vi "ge_EditCell.vi"(4 "HiLite":bool, 6 "Mod":bool, 7 "MeasType":T3, 8 "error in":errorcluster, 9 "Active Cell":T4, 10 "ge_DAQManDefinitions":T1, 11 "FP Ctrl":T2) -> (0 "error out":errorcluster, 1 "Discard?":bool)   [LabVIEW 2018]
uses:
  <vilib>/Utility/miscctls.llb/LVRowAndColumnTypeDef.ctl
  Custom Ctrls/ge_MeasType.ctl
  Custom Ctrls/ge_FPCtrlRefLabel.ctl
  Common/Controls/DAQMan Definitions.ctl
  Custom Ctls Table/ge_HdrInfo.ctl
  Custom Ctls Table/ge_GlblCtrls.ctl
  Custom Ctls Table/ge_ColType.ctl
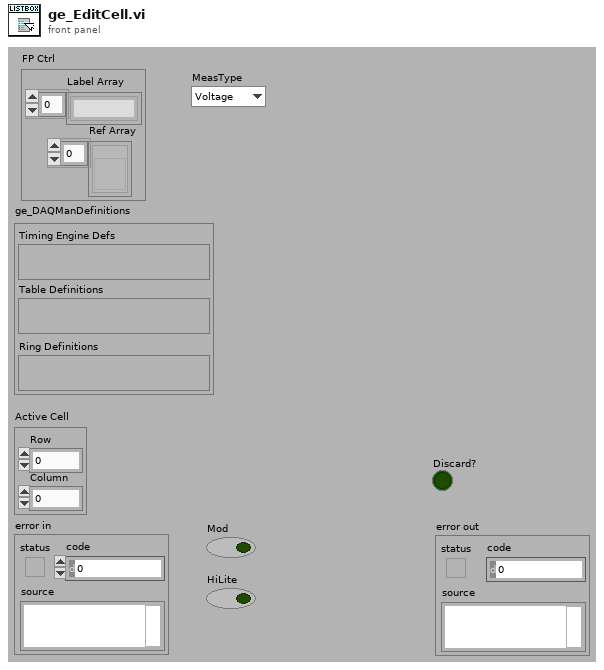
[diagram p1: front panel]
types:
  T1 = typedef "DAQMan Definitions.ctl" = cluster{"Timing Engine Defs":variant, "Table Definitions":variant, "Ring Definitions":variant}
  T2 = typedef "ge_FPCtrlRefLabel.ctl" = cluster{"Label Array":string[], "Ref Array":refnum<vi>[]}
  T3 = typedef "ge_MeasType.ctl" = enum16{"Voltage", "Frequency", "Tachometer", "Dynamic", "Thermocouple", "RTD", "Strain", "Current", "Resistance"}
  T4 = typedef "LVRowAndColumnTypeDef.ctl" = cluster{"Row":i32, "Column":i32}
  T5 = typedef "ge_HdrInfo.ctl" = cluster{"Hdr Width":i32, "Glbl Ctrl":T6}
  T6 = typedef "ge_GlblCtrls.ctl" = enum16{"Str0", "Bool0", "Bool1", "Int0", "Ring0", "Ring1", "Ring2", "Ring3", "Dbl0", "Dbl1", "Dbl2", "Dbl3", "Cal0", "Cal1", "Cal2", "None"}
  T7 = typedef "LVPositionTypeDef.ctl" = cluster{"Left":i32, "Top":i32}
  T8 = typedef "LVBoundsTypeDef.ctl" = cluster{"Width":u32, "Height":u32}
  T9 = typedef "ge_ColType.ctl" = enum16{"Volts", "Amps", "Ohms", "TermCfg", "WireCfg", "Coup", "Slope", "Iex", "CalUnits", "ThrmUnits", "ThrmType", "CJCSrc", "BrdgType", "Strn Mode", "RTDType"}
  T10 = typedef "HeaderNames.ctl" = enum16{"Channel", "Device", "Spacer", "Description", "MB", "Range", "Terminal", "Coupling", "Thresh (V)", "Pulse/Rev", "Slope", "Min EU", "Min RPM", "mV/EU", "Iex", "Temp Units", "Type", "CJC Src", "CJC Val", "Ro", "Wire Cfg", "Strain Mode", "Vex", "Bridge Type", "GF", "Gauge Res", "Poisson", "Lead Res", "Init Strain", "GAF", "Scale", "Offset", "Unit (EU)", "dB?", "dB Ref", "Cal Mag", "Cal Units", "Max Temp", "Min Temp", "Max Strain", "Min Strain"}
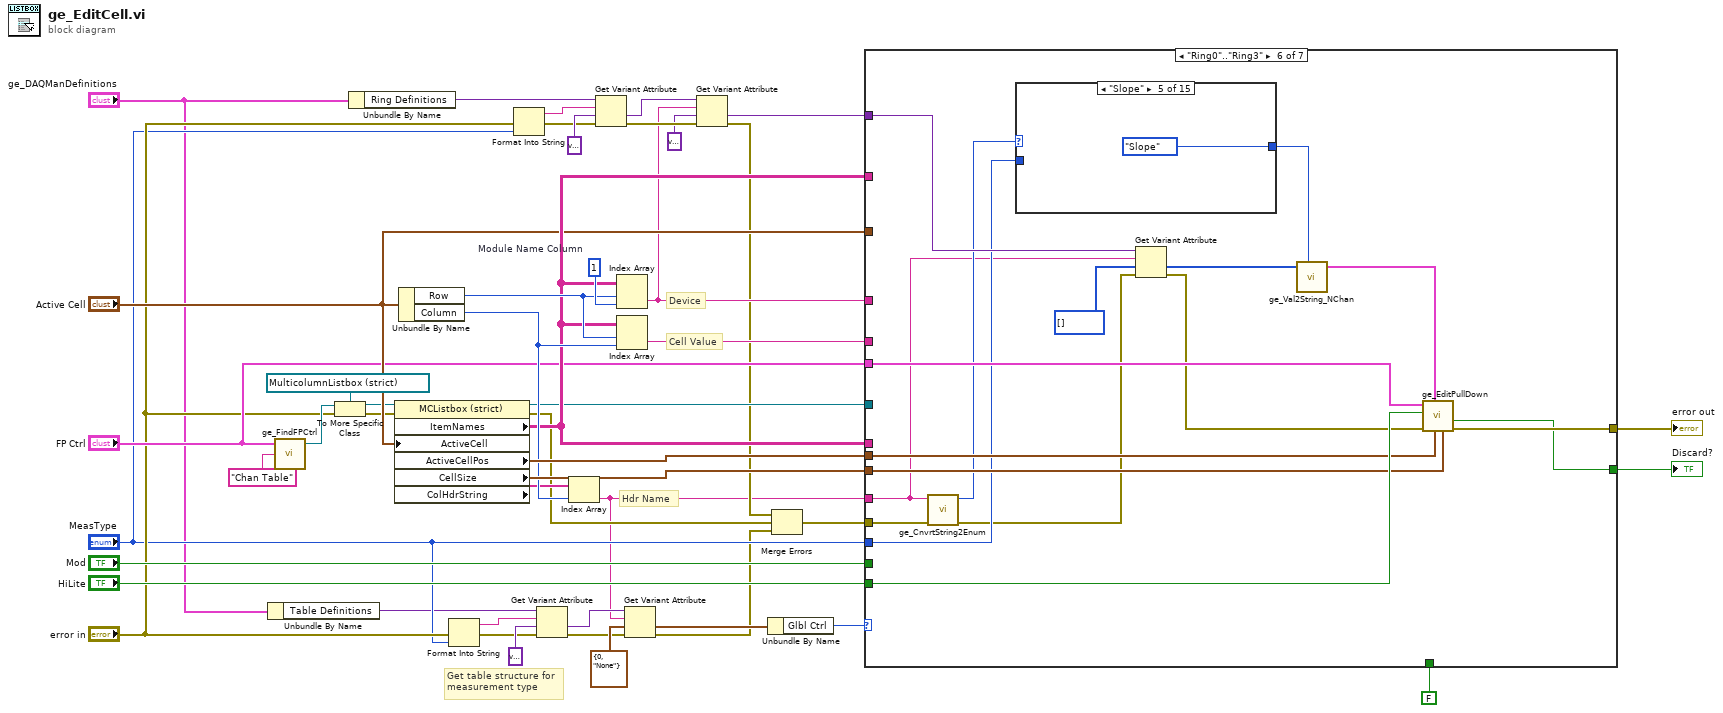
[diagram p0: block diagram]
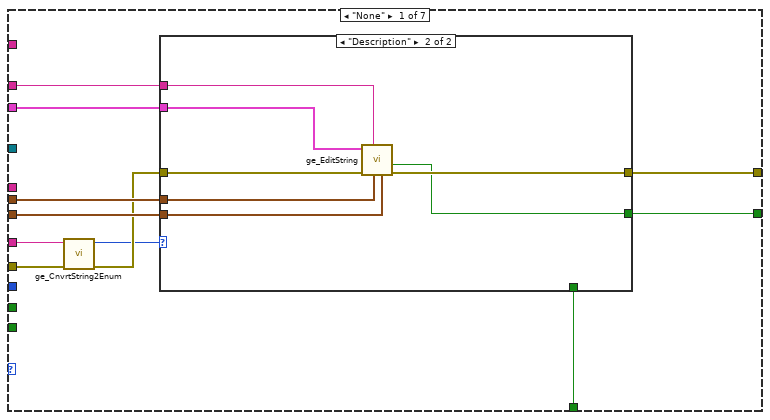
[diagram p2: hidden frame]
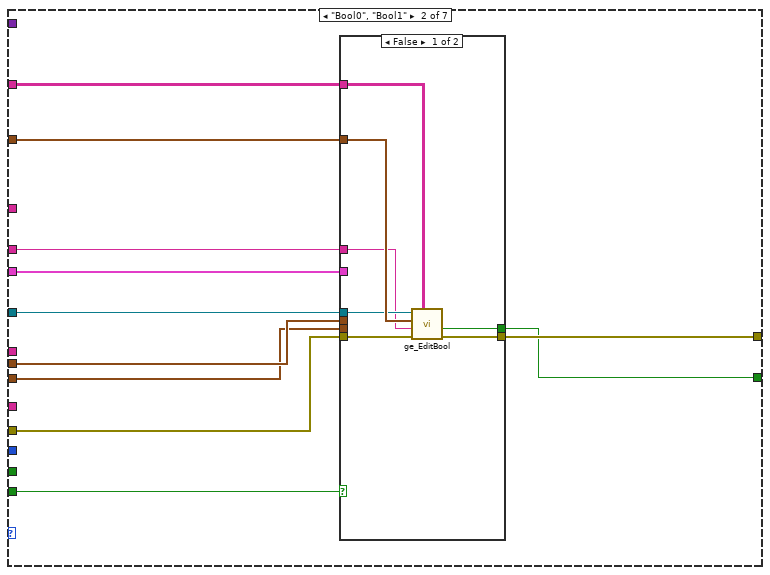
[diagram p4: hidden frame]
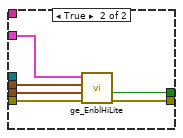
[diagram p5: hidden frame]
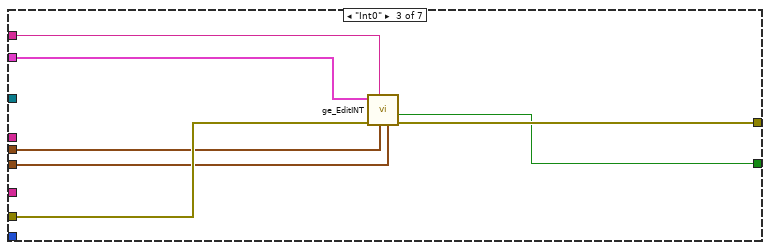
[diagram p6: hidden frame]
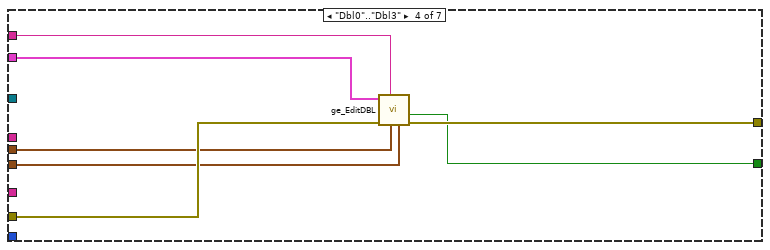
[diagram p7: hidden frame]
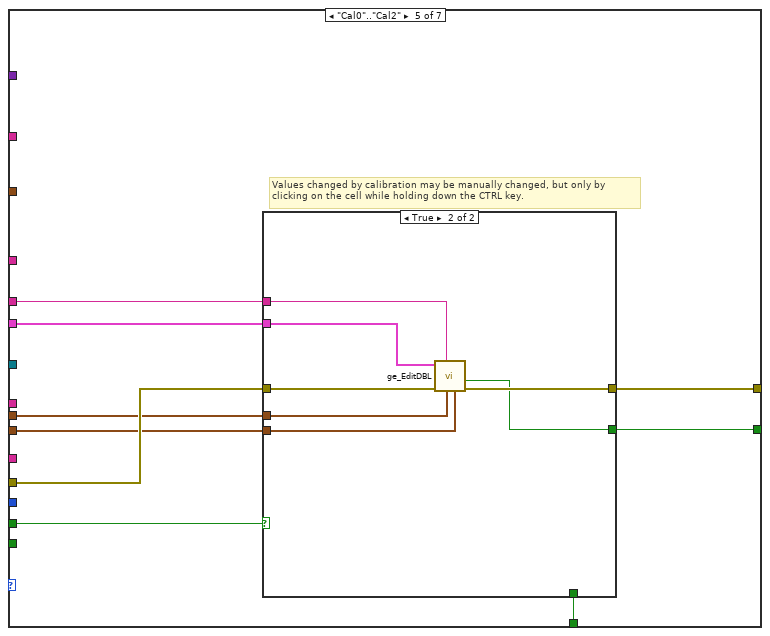
[diagram p8: hidden frame]
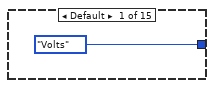
[diagram p10: hidden frame]
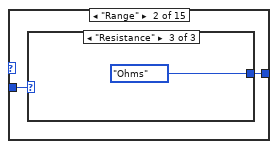
[diagram p11: hidden frame]
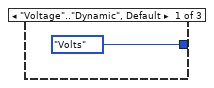
[diagram p12: hidden frame]
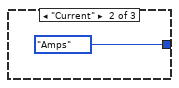
[diagram p13: hidden frame]
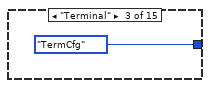
[diagram p14: hidden frame]
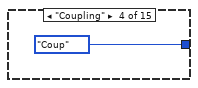
[diagram p15: hidden frame]
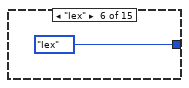
[diagram p16: hidden frame]
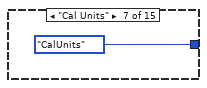
[diagram p17: hidden frame]
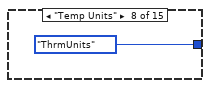
[diagram p18: hidden frame]
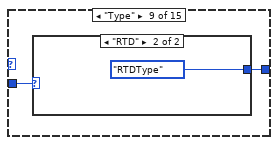
[diagram p19: hidden frame]
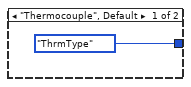
[diagram p20: hidden frame]
diagram:
  w47 = 1  # Module Name Column
  # "Get table structure for\nmeasurement type"
  # "Hdr Name"
  # "Cell Value"
  # "Device"
  n1 = Unbundle By Name("ge_DAQManDefinitions") -> ("Table Definitions"=w2:variant)
  n2 = call "ge_FindFPCtrl.vi"("Ctrl Name"="Chan Table" ("Name"), "FP Ctrl"="FP Ctrl") -> ("Ctrl Ref"=w36:refnum<vi>)  [unwired: 3 in]
  n3 = To More Specific Class(target class=refnum<vi> refnum ("reference"), reference=w36, error in="error in") -> (specific class reference=w34:refnum<vi>, error out=w33:errorcluster)
  n4 = Unbundle By Name("ge_DAQManDefinitions") -> ("Ring Definitions"=w3:variant)
  n5 = property class="MCListbox (strict)"(reference=w34, error in=w33, "ActiveCell"="Active Cell") -> (reference out=w31:refnum<vi>, error out=w5:errorcluster, "ItemNames"=w39:string[][], "ActiveCellPos"=w44:T7, "CellSize"=w43:T8, "ColHdrString"=w28:string[])
  n6 = Unbundle By Name("Active Cell") -> ("Row"=w42:i32, "Column"=w40:i32)
  n7 = Format Into String(error in="error in", "MeasType") -> (resulting string=w25:string, error out=w24:errorcluster)  [unwired: 2 in]
  n8 = Format Into String(error in="error in", "MeasType") -> (resulting string=w17:string, error out=w18:errorcluster)  [unwired: 2 in]
  n9 = Get Variant Attribute(Variant=w2, name=w25, default value (empty Variant)=variant ("All Ring Support"), error in=w24) -> (value=w23:variant, error out=w16:errorcluster)  [unwired: 2 out]
  n10 = Index Array(array=w28, index=w40) -> (element=w4:string)
  n11 = Get Variant Attribute(Variant=w3, name=w17, default value (empty Variant)=variant ("All Ring Support"), error in=w18) -> (value=w12:variant, error out=w13:errorcluster)  [unwired: 2 out]
  n12 = Index Array(array=w39, index (row)=w42, index (col)=w47) -> (element=w11:string)
  n13 = Index Array(array=w39, index (row)=w42, index (col)=w40) -> (element=w41:string)
  n14 = Get Variant Attribute(Variant=w23, name=w4, default value (empty Variant)=T5 {"Hdr Width"=0, "Glbl Ctrl"=enum."None"} ("HdrInfo"), error in=w16) -> (value=w21:T5, error out=w6:errorcluster)  [unwired: 2 out]
  n15 = Get Variant Attribute(Variant=w12, name=w11, default value (empty Variant)=variant ("All Ring Support"), error in=w13) -> (value=w9:variant, error out=w7:errorcluster)  [unwired: 2 out]
  n16 = Unbundle By Name(w21) -> ("Glbl Ctrl"=w20:T6)
  n17 = Merge Errors(w7, w5, w6) -> (w8:errorcluster)
  n18 = case shown="\"Ring0\"..\"Ring3\"" w20 {
    tunnel: w11 -> [_ _ _ _ _ _ _]
    tunnel: [w54 w77 w97 w104 w113 w138 w168] -> w46
    tunnel: [w53 w73 w94 w103 w112 w137 w167] -> w45
    tunnel: "MeasType" -> [_ _ _ _ _ w128 _]
    tunnel: w8 -> [w51 w78 w98 w105 w114 w127 w169]
    tunnel: w44 -> [w56 w75 w93 w100 w108 w134 w164]
    tunnel: "FP Ctrl" -> [w58 w76 w95 w101 w110 w135 w166]
    tunnel: w43 -> [w55 w74 w92 w99 w107 w133 w163]
    tunnel: w41 -> [w57 w68 w96 w102 w109 _ w165]
    tunnel: w39 -> [_ _ _ _ _ _ _]
    tunnel: w39 -> [_ w70 _ _ _ _ _]
    tunnel: "Active Cell" -> [_ w71 _ _ _ _ _]
    tunnel: w31 -> [_ w69 _ _ _ _ _]
    tunnel: "Mod" -> [_ _ _ _ w111 _ _]
    tunnel: "HiLite" -> [_ w72 _ _ _ w136 _]
    tunnel: FALSE ("Discard?") -> [w52 _ _ _ w106 _ _]
    tunnel: w9 -> [_ _ _ _ _ w131 _]
    tunnel: w4 -> [w49 _ _ _ _ w124 _]
    frame "None" {
      n19 = call "ge_CnvrtString2Enum.vi"("error in (no error)"=w51, "Enum String"=w49) -> ("error out"=w50:errorcluster, "Hdr Name"=w48:T10)  [unwired: 8 in]
      n20 = case shown="\"Description\"" w48 {
        tunnel: w50 -> [w60 w67]
        tunnel: w58 -> [_ w66]
        tunnel: w57 -> [_ w65]
        tunnel: w56 -> [_ w64]
        tunnel: w55 -> [_ w63]
        tunnel: [w60 w62] -> w54
        tunnel: [w59 w61] -> w53
        tunnel: w52 -> [w59 _]
        frame Default {
        }
        frame "Description" {
          n21 = call "ge_EditString.vi"("CellSize"=w63, "ActiveCellPos"=w64, "String"=w65, "error in"=w67, "FP Ctrl"=w66) -> ("error out"=w62:errorcluster, "Discard?"=w61:bool)  [unwired: 5 in]
        }
      }
    }
    frame "Bool0", "Bool1" {
      n22 = case shown="False" w72 {
        tunnel: w78 -> [w85 w91]
        tunnel: [w84 w90] -> w77
        tunnel: w76 -> [_ w89]
        tunnel: w75 -> [_ w88]
        tunnel: w74 -> [_ w87]
        tunnel: [w83 w86] -> w73
        tunnel: w71 -> [w82 _]
        tunnel: w70 -> [w81 _]
        tunnel: w69 -> [w80 _]
        tunnel: w68 -> [w79 _]
        frame False {
          n23 = call "ge_EditBool.vi"("ItemNames"=w81, "error in"=w85, "Cell Val"=w79, "Active Cell"=w82, "reference"=w80) -> ("error out"=w84:errorcluster, "Discard?"=w83:bool)  [unwired: 5 in]
        }
        frame True {
          n24 = call "ge_EnblHiLite.vi"("error in"=w91, "CellSize"=w87, "ActiveCellPos"=w88, "FP Ctrl"=w89) -> ("error out"=w90:errorcluster, "Discard?"=w86:bool)  [unwired: 6 in]
        }
      }
    }
    frame "Int0" {
      n25 = call "ge_EditINT.vi"("CellSize"=w92, "ActiveCellPos"=w93, "String Value"=w96, "error in"=w98, "FP Ctrl"=w95) -> ("error out"=w97:errorcluster, "Discard?"=w94:bool)  [unwired: 5 in]
    }
    frame "Dbl0".."Dbl3" {
      n26 = call "ge_EditDBL.vi"("CellSize"=w99, "ActiveCellPos"=w100, "String Value"=w102, "error in"=w105, "FP Ctrl"=w101) -> ("error out"=w104:errorcluster, "Discard?"=w103:bool)  [unwired: 5 in]
    }
    frame "Cal0".."Cal2" {
      # "Values changed by calibration may be manually changed, but only by\nclicking on the cell while holding down the CTRL key."
      n27 = case shown="True" w111 {
        tunnel: w114 -> [w116 w123]
        tunnel: [w116 w122] -> w113
        tunnel: [w115 w121] -> w112
        tunnel: w110 -> [_ w120]
        tunnel: w109 -> [_ w119]
        tunnel: w108 -> [_ w118]
        tunnel: w107 -> [_ w117]
        tunnel: w106 -> [w115 _]
        frame False {
        }
        frame True {
          n28 = call "ge_EditDBL.vi"("CellSize"=w117, "ActiveCellPos"=w118, "String Value"=w119, "error in"=w123, "FP Ctrl"=w120) -> ("error out"=w122:errorcluster, "Discard?"=w121:bool)  [unwired: 5 in]
        }
      }
    }
    frame "Ring0".."Ring3" {
      n29 = call "ge_CnvrtString2Enum.vi"("error in (no error)"=w127, "Enum String"=w124) -> ("error out"=w126:errorcluster, "Hdr Name"=w125:T10)  [unwired: 8 in]
      n30 = case shown="\"Slope\"" w125 {
        tunnel: [ge_ColType."Volts" ("ColType") w143 ge_ColType."TermCfg" ("ColType") ge_ColType."Coup" ("ColType") ge_ColType."Slope" ("ColType") ge_ColType."Iex" ("ColType") ge_ColType."CalUnits" ("ColType") ge_ColType."ThrmUnits" ("ColType") w153 ge_ColType."CJCSrc" ("ColType") ge_ColType."Ohms" ("ColType") ge_ColType."WireCfg" ("ColType") ge_ColType."Strn Mode" ("ColType") ge_ColType."Volts" ("ColType") ge_ColType."BrdgType" ("ColType")] -> w139
        tunnel: w128 -> [_ w142 _ _ _ _ _ _ w154 _ _ _ _ _ _]
        frame Default {
        }
        frame "Range" {
          n31 = case shown="\"Resistance\"" w142 {
            tunnel: [ge_ColType."Volts" ("ColType") ge_ColType."Amps" ("ColType") ge_ColType."Ohms" ("ColType")] -> w143
            frame "Voltage".."Dynamic", Default {
            }
            frame "Current" {
            }
            frame "Resistance" {
            }
          }
        }
        frame "Terminal" {
        }
        frame "Coupling" {
        }
        frame "Slope" {
        }
        frame "Iex" {
        }
        frame "Cal Units" {
        }
        frame "Temp Units" {
        }
        frame "Type" {
          n32 = case shown="\"RTD\"" w154 {
            tunnel: [ge_ColType."ThrmType" ("ColType") ge_ColType."RTDType" ("ColType")] -> w153
            frame "Thermocouple", Default {
            }
            frame "RTD" {
            }
          }
        }
        frame "CJC Src" {
        }
        frame "Ro" {
        }
        frame "Wire Cfg" {
        }
        frame "Strain Mode" {
        }
        frame "Vex" {
        }
        frame "Bridge Type" {
        }
      }
      n33 = Get Variant Attribute(Variant=w131, name=w124, default value (empty Variant)=u16[] [] ("Values"), error in=w126) -> (value=w129:u16[], error out=w130:errorcluster)  [unwired: 2 out]
      n34 = call "ge_Val2String_NChan.vi"("Values"=w129, "ColType"=w139) -> ("String and Values"=w140:cluster{"String":string, "Value":u16}[])  [unwired: 5 in]
      n35 = call "ge_EditPullDown.vi"("CellSize"=w133, "ActiveCellPos"=w134, "String and Values"=w140, "error in"=w130, "PD HiLite"=w136, "FP Ctrl"=w135) -> ("error out"=w138:errorcluster, "Discard?"=w137:bool)  [unwired: 4 in]
    }
    frame "Str0" {
      n36 = call "ge_EditString.vi"("CellSize"=w163, "ActiveCellPos"=w164, "String"=w165, "error in"=w169, "FP Ctrl"=w166) -> ("error out"=w168:errorcluster, "Discard?"=w167:bool)  [unwired: 5 in]
    }
  }
  "error out" <- w46
  "Discard?" <- w45
